vi "io_rotate_around_principal_axis.vi"(5 "mode":T1, 7 "axis":T2, 8 "error in (no error)":errorcluster, 10 "angle":dbl[unit], 11 "points in":dbl[][](array[numeric])) -> (0 "error out":errorcluster, 3 "points out":dbl[][](array[numeric]))   [LabVIEW 2010, in "PointCollection.lvclass"]
uses:
  PointCollection.lvclass
  x_y_z_enumeration.ctl
  mode_enum.ctl
  <vilib>/Analysis/Matrix/Numeric/Conversions/Array To Matrix - RA2.vi
  <vilib>/Analysis/baseanly.llb/Real A x B.vi
  <vilib>/Analysis/Matrix/NI_Matrix.lvlib
  <vilib>/Analysis/NI_AALBase.lvlib
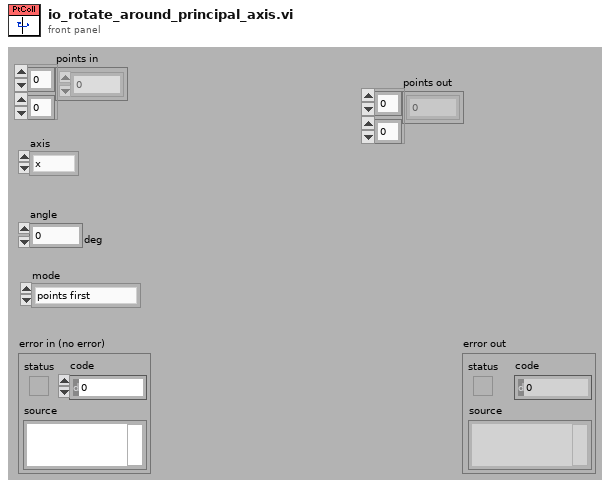
[diagram p1: front panel]
types:
  T1 = typedef "PointCollection.lvclass/mode_enum.ctl" = enum16{"points first", "dimensions first"}
  T2 = typedef "PointCollection.lvclass/x_y_z_enumeration.ctl" = enum16{"x", "y", "z"}
  T3 = typedef "NI_Matrix.lvlib/RealMatrix.ctl" = dbl[][]
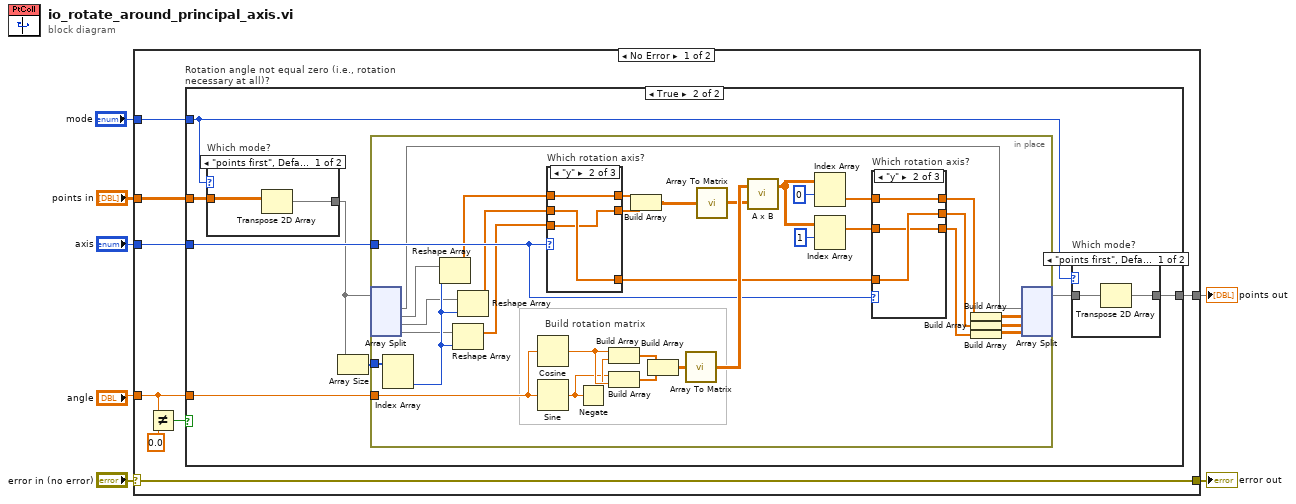
[diagram p0: block diagram]
diagram:
  n1 = case shown="No Error" "error in (no error)" {
    selector: "error in (no error)" -> [w10 w83]
    tunnel: [w10 w83] -> w7
    tunnel: "angle" -> [w13 _]
    tunnel: "axis" -> [w12 _]
    tunnel: [w11 _] -> w2
    tunnel: "points in" -> [w9 _]
    tunnel: "mode" -> [w8 _]
    frame No Error {
      n2 = Not Equal?(x=w13, y=dbl[unit] 0.0) -> (x != y?=w14:bool)
      n3 = case "Rotation angle not equal zero (i.e., rotation necessary at all)?" shown="True" w14 {
        tunnel: w13 -> [_ w24]
        tunnel: w12 -> [_ w23]
        tunnel: [w16 w18] -> w11
        tunnel: w9 -> [w16 w21]
        tunnel: w8 -> [_ w17]
        frame False {
        }
        frame True {
          n4 = case "Which mode?" shown="\"points first\", Default" w17 {
            tunnel: w21 -> [w29 w30]
            tunnel: [w28 w30] -> w20
            frame "points first", Default {
              n5 = Transpose 2D Array(2D array=w29) -> (transposed array=w28:dbl[][])
            }
            frame "dimensions first" {
            }
          }
          n6 = Array Size(array=w20) -> (size(s)=w22:i32[])
          n7 = in-place {
            in-place-border: w24 -> [w50]
            in-place-border: w23 -> [w49]
            in-place-border: w22 -> [w39]
            # "Build rotation matrix"
            n8 = in-place-split #1(w20) -> (w31:dbl[][], w35:dbl[][], w36:dbl[][], w37:dbl[][])  [unwired: 3 in]
            n9 = Index Array(array=w39) -> (element #2=w38:i32)  [unwired: 2 in, 1 out]
            n10 = Reshape Array(w35, w38) -> (w45:dbl[])
            n11 = Reshape Array(w37, w38) -> (w43:dbl[])
            n12 = Reshape Array(w36, w38) -> (w44:dbl[])
            n13 = Cosine(x=w50) -> (cos(x)=w61:dbl)
            n14 = Sine(x=w50) -> (sin(x)=w59:dbl)
            n15 = case "Which rotation axis?" shown="\"y\"" w49 {
              tunnel: [w75 w78 w82] -> w54
              tunnel: w45 -> [w76 w78 w82]
              tunnel: [w74 w77 w81] -> w53
              tunnel: w44 -> [w75 w79 w81]
              tunnel: [w76 w79 w80] -> w51
              tunnel: w43 -> [w74 w77 w80]
              frame "x", Default {
              }
              frame "y" {
              }
              frame "z" {
              }
            }
            n16 = Negate(x=w59) -> (-x=w60:dbl)
            n17 = Build Array(w61, w60) -> (w64:dbl[])
            n18 = Build Array(w59, w61) -> (w63:dbl[])
            n19 = Build Array(w54, w53) -> (w46:dbl[][])
            n20 = Build Array(w64, w63) -> (w62:dbl[][])
            n21 = call-poly <vilib>:"Array To Matrix.vi"("Real 2D Array"=w62) -> ("Real Matrix"=w55:T3)
            n22 = call-poly <vilib>:"Array To Matrix.vi"("Real 2D Array"=w46) -> ("Real Matrix"=w52:T3)
            n23 = call-poly <vilib>:"A x B.vi"("B"=w52, "A"=w55) -> ("A x B"=w56:T3)  [unwired: 1 out]
            n24 = Index Array(array=w56, index (row)=0) -> (element=w48:dbl[])  [unwired: 1 in]
            n25 = Index Array(array=w56, index (row)=1) -> (element=w47:dbl[])  [unwired: 1 in]
            n26 = case "Which rotation axis?" shown="\"y\"" w49 {
              tunnel: [w67 w69 w73] -> w42
              tunnel: w48 -> [w66 w69 w73]
              tunnel: [w66 w70 w72] -> w41
              tunnel: w47 -> [w65 w68 w72]
              tunnel: [w65 w68 w71] -> w40
              tunnel: w51 -> [w67 w70 w71]
              frame "x", Default {
              }
              frame "y" {
              }
              frame "z" {
              }
            }
            n27 = Build Array(w42) -> (w32:dbl[][])
            n28 = Build Array(w41) -> (w33:dbl[][])
            n29 = Build Array(w40) -> (w34:dbl[][])
            n30 = in-place-split #1(w31, w32, w33, w34) -> (w19:dbl[][])  [unwired: 3 out]
          }
          n31 = case "Which mode?" shown="\"points first\", Default" w17 {
            tunnel: w19 -> [w26 w27]
            tunnel: [w25 w27] -> w18
            frame "points first", Default {
              n32 = Transpose 2D Array(2D array=w26) -> (transposed array=w25:dbl[][])
            }
            frame "dimensions first" {
            }
          }
        }
      }
    }
    frame Error {
    }
  }
  "error out" <- w7
  "points out" <- w2
